vi "去除数组无效0.vi"(10 "数值":i32, 11 "数组":dbl[](array[numeric])) -> (3 "数组 2":dbl[](array[numeric]))   [LabVIEW 2021]
uses:
  b2582d41-7725-432c-8ed4-e69de8133079.vi
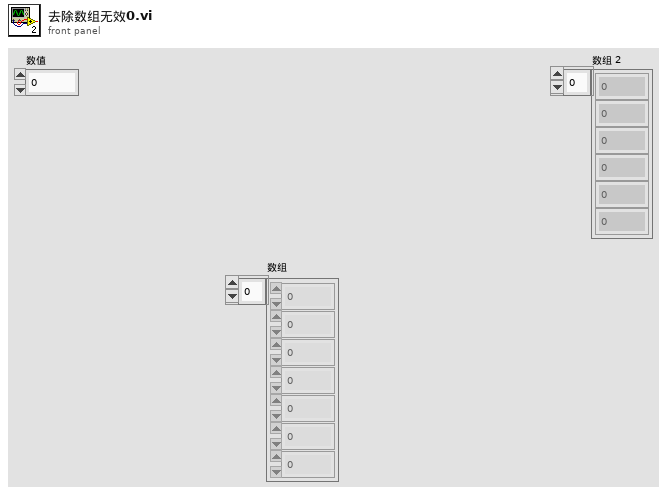
[diagram p1: front panel]
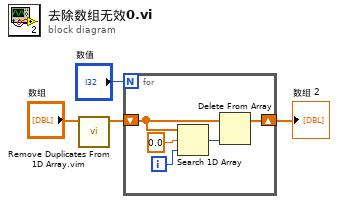
[diagram p0: block diagram]
diagram:
  n1 = call "Remove Duplicates From 1D Array.vim"("array"="数组") -> ("array with duplicates removed"=w1:dbl[])  [unwired: 10 in]
  n2 = for {
    N: "数值" -> [_]
    shift-right: [w7] -> w3
    shift-left: w1 -> [w6]
    i -> [w9]
    n3 = Search 1D Array(1D array=w6, element=0.0 ("元素"), start index (0)=w9) -> (index of element=w8:i32)
    n4 = Delete From Array(array=w6, index=w8) -> (array with subset deleted=w7:dbl[])  [unwired: 1 in, 1 out]
  }
  "数组 2" <- w3
